vi "2 line cross point.vi"(1 "D":cluster{dbl, dbl}, 2 "C":cluster{dbl, dbl}, 3 "B":cluster{dbl, dbl}, 4 "A":cluster{dbl, dbl}) -> (0 "cross center":cluster{dbl, dbl})   [LabVIEW 2019]
panel:
  out "XY Graph":cluster{cluster{dbl, dbl}[]}[](graph)
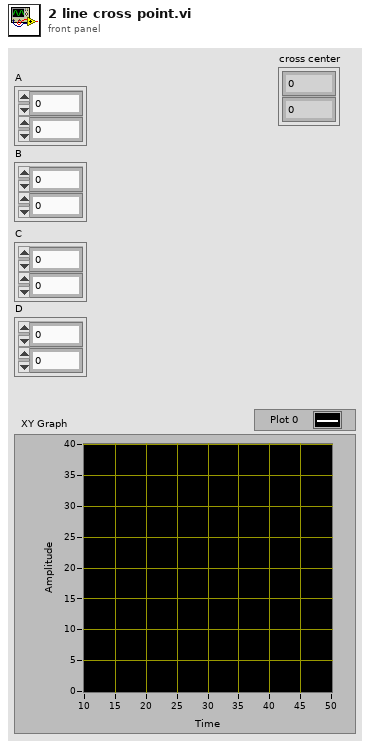
[diagram p1: front panel]
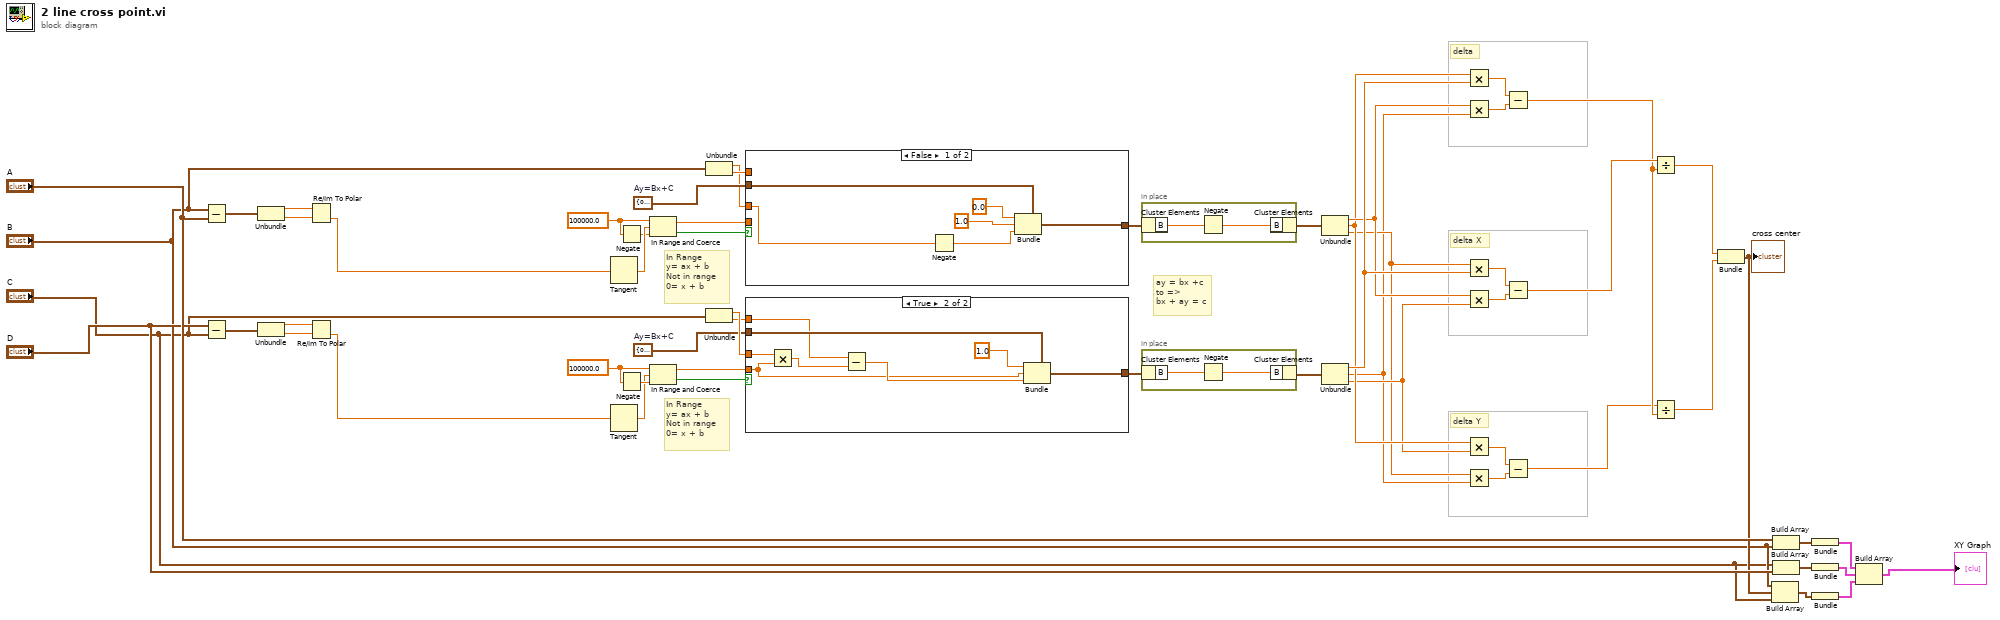
[diagram p0: block diagram]
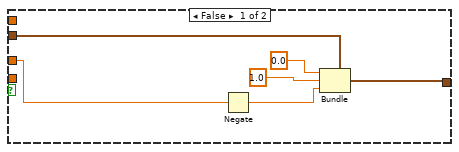
[diagram p2: hidden frame]
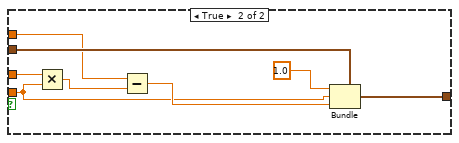
[diagram p3: hidden frame]
diagram:
  w36 = 100000.0
  w39 = cluster{"A":dbl, "B":dbl, "C":dbl} {"A"=0.0, "B"=0.0, "C"=0.0}  # Ay=Bx+C
  w50 = 100000.0
  w47 = cluster{"A":dbl, "B":dbl, "C":dbl} {"A"=0.0, "B"=0.0, "C"=0.0}  # Ay=Bx+C
  # "delta Y"
  # "delta X"
  # "delta"
  # "ay = bx +c \nto =>\nbx + ay = c"
  # "In Range \ny= ax + b\nNot in range\n0= x + b"
  # "In Range \ny= ax + b\nNot in range\n0= x + b"
  n1 = Subtract(x="B", y="A") -> (x-y=w46:cluster{dbl, dbl})
  n2 = Subtract(x="D", y="C") -> (x-y=w57:cluster{dbl, dbl})
  n3 = Unbundle(w46) -> (w56:dbl, w55:dbl)
  n4 = Unbundle(w57) -> (w54:dbl, w53:dbl)
  n5 = Re/Im To Polar(2:w55, 3:w56) -> (0:w52:dbl)  [unwired: 1 out]
  n6 = Re/Im To Polar(2:w53, 3:w54) -> (0:w13:dbl)  [unwired: 1 out]
  n7 = Tangent(1:w52) -> (0:w51:dbl)
  n8 = Tangent(1:w13) -> (0:w35:dbl)
  n9 = Negate(x=w50) -> (-x=w49:dbl)
  n10 = Negate(x=w36) -> (-x=w37:dbl)
  n11 = In Range and Coerce(upper limit=w50, x=w51, lower limit=w49) -> (coerced(x)=w44:dbl, In Range?=w48:bool)
  n12 = In Range and Coerce(upper limit=w36, x=w35, lower limit=w37) -> (coerced(x)=w41:dbl, In Range?=w38:bool)
  n13 = Unbundle("B") -> (w43:dbl, w45:dbl)
  n14 = Unbundle("C") -> (w42:dbl, w40:dbl)
  n15 = case shown="False" w48 {
    tunnel: w47 -> [w63 w71]
    tunnel: w45 -> [_ w69]
    tunnel: w44 -> [_ w65]
    tunnel: w43 -> [w59 w68]
    tunnel: [w58 w64] -> w34
    frame False {
      n16 = Negate(x=w59) -> (-x=w60:dbl)
      n17 = Bundle(cluster=w63, "A"=0.0, "B"=1.0, "C"=w60) -> (w58:cluster{"A":dbl, "B":dbl, "C":dbl})
    }
    frame True {
      n18 = Multiply(x=w68, y=w65) -> (x*y=w67:dbl)
      n19 = Subtract(x=w69, y=w67) -> (x-y=w66:dbl)
      n20 = Bundle(cluster=w71, "A"=1.0, "B"=w65, "C"=w66) -> (w64:cluster{"A":dbl, "B":dbl, "C":dbl})
    }
  }
  n21 = case shown="True" w38 {
    tunnel: w39 -> [w77 w85]
    tunnel: w40 -> [_ w83]
    tunnel: w41 -> [_ w79]
    tunnel: w42 -> [w73 w82]
    tunnel: [w72 w78] -> w33
    frame False {
      n22 = Negate(x=w73) -> (-x=w74:dbl)
      n23 = Bundle(cluster=w77, "A"=0.0, "B"=1.0, "C"=w74) -> (w72:cluster{"A":dbl, "B":dbl, "C":dbl})
    }
    frame True {
      n24 = Multiply(x=w82, y=w79) -> (x*y=w81:dbl)
      n25 = Subtract(x=w83, y=w81) -> (x-y=w80:dbl)
      n26 = Bundle(cluster=w85, "A"=1.0, "B"=w79, "C"=w80) -> (w78:cluster{"A":dbl, "B":dbl, "C":dbl})
    }
  }
  n27 = in-place {
    n28 = in-place-cluster #1(w34) -> ("B"=w87:dbl)
    n29 = Negate(x=w87) -> (-x=w86:dbl)
    n30 = in-place-cluster #1("B"=w86) -> (w32:cluster{"A":dbl, "B":dbl, "C":dbl})
  }
  n31 = in-place {
    n32 = in-place-cluster #2(w33) -> ("B"=w89:dbl)
    n33 = Negate(x=w89) -> (-x=w88:dbl)
    n34 = in-place-cluster #2("B"=w88) -> (w31:cluster{"A":dbl, "B":dbl, "C":dbl})
  }
  n35 = Unbundle(w32) -> ("A"=w23:dbl, "B"=w22:dbl, "C"=w20:dbl)
  n36 = Unbundle(w31) -> ("A"=w26:dbl, "B"=w19:dbl, "C"=w21:dbl)
  n37 = Multiply(x=w22, y=w26) -> (x*y=w30:dbl)
  n38 = Multiply(x=w23, y=w19) -> (x*y=w29:dbl)
  n39 = Multiply(x=w20, y=w26) -> (x*y=w27:dbl)
  n40 = Multiply(x=w23, y=w21) -> (x*y=w28:dbl)
  n41 = Multiply(x=w22, y=w21) -> (x*y=w25:dbl)
  n42 = Multiply(x=w20, y=w19) -> (x*y=w24:dbl)
  n43 = Subtract(x=w30, y=w29) -> (x-y=w17:dbl)
  n44 = Subtract(x=w27, y=w28) -> (x-y=w18:dbl)
  n45 = Subtract(x=w25, y=w24) -> (x-y=w16:dbl)
  n46 = Divide(x=w18, y=w17) -> (x/y=w15:dbl)
  n47 = Divide(x=w16, y=w17) -> (x/y=w14:dbl)
  n48 = Bundle(w15, w14) -> (w8:cluster{dbl, dbl})  [unwired: 1 in]
  "cross center" <- w8
  n49 = Build Array("B", w8, "C") -> (w5:cluster{dbl, dbl}[])
  n50 = Build Array("A", "B") -> (w10:cluster{dbl, dbl}[])
  n51 = Build Array("C", "D") -> (w9:cluster{dbl, dbl}[])
  n52 = Bundle(w10) -> (w4:cluster{cluster{dbl, dbl}[]})  [unwired: 1 in]
  n53 = Bundle(w9) -> (w3:cluster{cluster{dbl, dbl}[]})  [unwired: 1 in]
  n54 = Bundle(w5) -> (w2:cluster{cluster{dbl, dbl}[]})  [unwired: 1 in]
  n55 = Build Array(w4, w3, w2) -> (→"XY Graph":cluster{cluster{dbl, dbl}[]}[])
